vi "Actor Core.vi"(8 "error in (no error)":errorcluster, 11 "CalibrationManagerActor.lvlib:CalibrationManagerActor.lvclass":refnum<class "CalibrationManagerActor.lvclass">) -> (0 "error out":errorcluster, 3 "Actor out":refnum<class "Actor.lvclass">)   [LabVIEW 2017, in "CalibrationManagerActor.lvlib" / "CalibrationManagerActor.lvclass"]
doc: "This VI allows the user to view and edit instrument calibration details."
uses:
  CalibrationManagerActor.lvclass
  Library/SAM Resources 2.0/Main GUI/TSCalMan.llb/CalManData.ctl
  Library/SAM Resources 2.0/Main GUI/TSCalMan.llb/CalDataUnit.ctl
  <vilib>/ActorFramework/Actor/Actor.lvclass
  C:/Program Files (x86)/National Instruments/LabVIEW 2017/vi.lib/ActorFramework/Actor/Actor.lvclass
  SAMLite_DB/DB_Collections_class/mode.ctl
  CalibrationManagerActor.lvclass/CalibrationManagerActor.ctl
  Library/SAM Resources 2.0/Main GUI/TSCalMan.llb/CalMStates.ctl
  <vilib>/ActorFramework/Actor/Actor.lvclass/Actor.ctl
  <vilib>/ActorFramework/Message Enqueuer/Message Enqueuer.lvclass/Message Enqueuer.ctl
  <vilib>/ActorFramework/Message Enqueuer/Init from Existing Queue.vi
  <vilib>/ActorFramework/Message Enqueuer/Enqueue.vi
  <vilib>/ActorFramework/Stop Msg/Stop Msg.lvclass
  C:/Program Files (x86)/National Instruments/LabVIEW 2017/vi.lib/ActorFramework/Message/Message.lvclass
  <vilib>/ActorFramework/Message Priority Queue/Priority Enqueue.vi
  <vilib>/ActorFramework/Message Enqueuer/Message Enqueuer.lvclass
  GUI/GUI/GUI.lvclass
  Library/SAM Resources 2.0/Main GUI/SAMLite_Calibration Managemer.lvlib
  Library/SAM Resources 2.0/Main GUI/TestExec-STAC.llb/Full UI - Globals.vi
  Library/Amfax Library/Amfax Library/AmFax Source Code.lvclass
  SAMLite_DB/DB_Collections_class/DB_Collections.lvclass
  Library/Amfax Library/AmFax Source Code.lvlib
panel:
  in  "Edit Data File":bool
  in  "Calibration Data File":path
  in  "Alias Name":string
  out "Message":string
  in  "Cal Date Enabled":bool
  in  "Counter Enabled":bool
  in  "Calibration\n Interval":u32(ring) items=["Select an interval"=0, "1 month"=1, "2 months"=2, "6 months"=6, "12 months"=12, "24 months"=24]
  out "Current Count":u16=28 min=28 max=730 step=1
  in  "Total Cycles":i32
  in  "Cnt Warning":u16=28
  out "Traffic Light":cluster{"Red":bool, "Amber":bool, "Green":bool} caption="Calibration Status"
  in  "Reset Counter":bool
  in  "Cancel":bool
  in  "OK":bool
  in  "Cal Warning":u16=28
  in  "Type":string(combo)
  in  "Calibrated On":timestamp format="%<%x>T"
  in  "Cal Due Date":timestamp format="%<%x>T"
  in  "Cal":i32(listbox)
  out "Cal Expiry":u16=28 caption="Duration of\nCalibration" min=28 max=730 step=1
  in  "Clear All":bool
  in  "Delete":bool
  in  "Serial Number":string
  in  "Description":string
  in  "Update":bool
  in  "Add":bool
  in  "Cal Data FileName":string="CalInfo.bin"
  out "Cancelled":bool
  out "Calibration Out":T1 {"Cal Data Listing"."Cal Date" format="%<%x>T"; "Cal Data Listing"."Cal Due" format="%<%x>T"}
  out "Calibration Data Original":T1 {"Cal Data Listing"."Cal Date" format="%<%x>T"; "Cal Data Listing"."Cal Due" format="%<%x>T"}
  out "Out of Cal":bool
  # "Calibration Manager"
  # "Issue a Warning Message Ahead of Cycle Count by"
  # "Cycles"
  # "Days"
  # "Issue a Warning Message Ahead of Calibration Expiry Dates by"
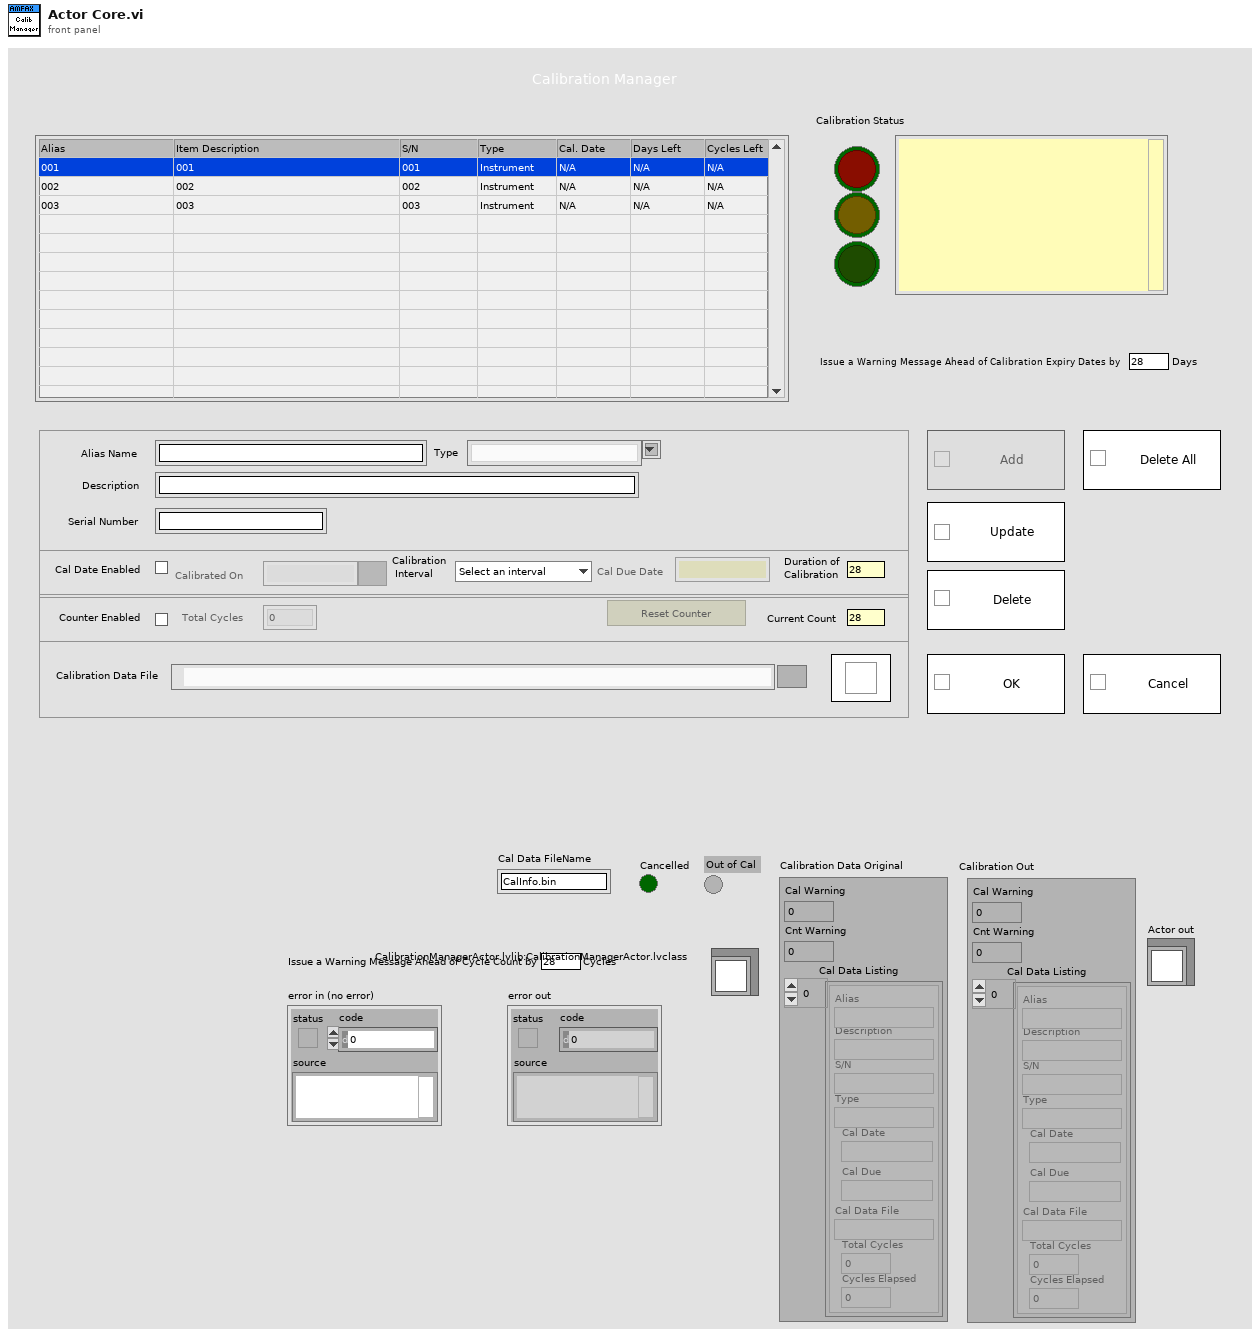
[diagram p1: front panel]
types:
  T1 = typedef "SAMLite_Calibration Managemer.lvlib/CalManData.ctl" = cluster{"Cal Warning":u32, "Cnt Warning":u16, "Cal Data Listing":T2[]}
  T2 = typedef "SAMLite_Calibration Managemer.lvlib/CalDataUnit.ctl" = cluster{"Alias":string, "Description":string, "S/N":string, "Type":string, "Cal Date":timestamp, "Cal Due":timestamp, "Cal Data File":path, "Total Cycles":i32, "Cycles Elapsed":i32}
  T3 = typedef "SAMLite_DB.lvlib/DB_Collections.lvclass/mode.ctl" = enum16{"read from file", "write to file", "set Defaults"}
  T4 = typedef "SAMLite_DB.lvlib/DB_Collections.lvclass/SAMLite Database.ctl" = cluster{"User Management":T5, "File Paths":cluster{"Path of test modules":path, "Path of sequences":path, "Path of test reports":path, "Path of Error Report":path, "Path of Calibration Data File":path, "Path of Company Logo":path, "Path of Startup VIs":path}, "Version Info":cluster{"Version No.":string}, "GUI Configuration":T8, "TARTCS_Intrument Control":T9, "Step Module Data":T17}
  T5 = typedef "SAMLite_DB.lvlib/DB_User.lvclass/User Management.ctl" = cluster{"Current User":string, "Current user group":T6, "Registered Users":cluster{"First Name":string, "Last Name":string, "User Name":string, "Password":string, "User Group":T6}[], "User Groups":cluster{"User Group":T6, "Members":string[], "User Previleges":T7}[]}
  T6 = typedef "SAMLite_DB.lvlib/DB_User.lvclass/User Group.ctl" = enum16{"Administrator", "Engineer", "Operator", "Data Viewer"}
  T7 = typedef "SAMLite_DB.lvlib/DB_User.lvclass/User Previleges.ctl" = cluster{"Run Sequences":bool, "Set Station Options":bool, "Instrument Configurations":bool, "Calibration Management":bool, "Access Test Reports Screen":bool, "Edit Test Sequences":bool, "Edit User":bool, "Add User":bool, "Delete User":bool, "Manual Control":bool, "Initialise System":bool}
  T8 = typedef "SAMLite_DB.lvlib/DB_SoftConfig.lvclass/GUI_Configurations.ctl" = cluster{"Main screen button caption color":u32, "Main screen display setting":enum32{"Modal", "Floating"}, "Debug Mode?":bool}
  T9 = typedef "SAMLite_DB.lvlib/DB_Collections.lvclass/TARTCS_InstrumentsSettings.ctl" = cluster{"Boom":T10, "Turntable":T13, "Inclinometer":T14, "Signal Generator Settings":cluster{"Resource Name (GPIB::28)":string}, "Spectrum Analyser Settings":cluster{"Resource Name (GPIB::28)":string}, "cRIO IP address":cluster{"Resource Name (GPIB::28)":string}}
  T10 = typedef "StreamComms.lvlib/Boom_Params.ctl" = cluster{"Master Node detail ":T11, "Slave Node Detail":T11, "Angle":dbl, "Motor Frequency %":dbl, "Max Leg Angle Difference":dbl, "Max Inclinometer to To Boom Leg  Angle Difference":dbl, "Angle Limits":cluster{"Max Operating Position":dbl, "Home Max Offset":dbl, "Home Position":dbl, "Home Min Offset":dbl, "Min Operating Position":dbl}, "Step Angle":dbl, "Select Boom/Inc Trigger":enum16{"Inclinometer", "Boom"}}
  T11 = typedef "StreamComms.lvlib/Inverter_NodeInfo.ctl" = cluster{"Node ID":u8, "baud rate":T12, "termination required? (F)":bool, "interface name":u32, "Inverter Name":string}
  T12 = typedef "CANopen BaudRate.ctl" = u32
  T13 = typedef "StreamComms.lvlib/Turntable_Params.ctl" = cluster{"Node Detail":T11, "Angle":dbl, "Motor Frequency %":dbl, "Trigger Step Angle":dbl}
  T14 = typedef "StreamComms.lvlib/Inclinometer_Params.ctl" = cluster{"Node Detail":T15, "filter cutoff (milli Hz)":dbl, "Triger angle":dbl, "Zero Offset (deg)":dbl}
  T15 = typedef "StreamComms.lvlib/CANOpen_NodeDetail.ctl" = cluster{"LSS Identity Details":T16, "Node ID":u8, "baud rate":T12, "termination required? (F)":bool, "interface name":u32}
  T16 = typedef "StreamComms.lvlib/CANOpen LSS Identity.ctl" = cluster{"Vendor ID":u32, "Product Code":u32, "Revision Number":u32, "Serial Number":u32}
  T17 = typedef "SAMLite_DB.lvlib/DB_StepModule.lvclass/Step Module Date.ctl" = cluster{"Error Out":errorcluster}
  T18 = enum8{"Enabled", "Disabled", "Disabled and Grayed Out"}
  T19 = typedef "CalibrationManagerActor.lvlib/CalibrationManagerActor.lvclass/CalMStates.ctl" = enum16{"Initialise", "Event", "Screen Update", "Save", "Exit"}
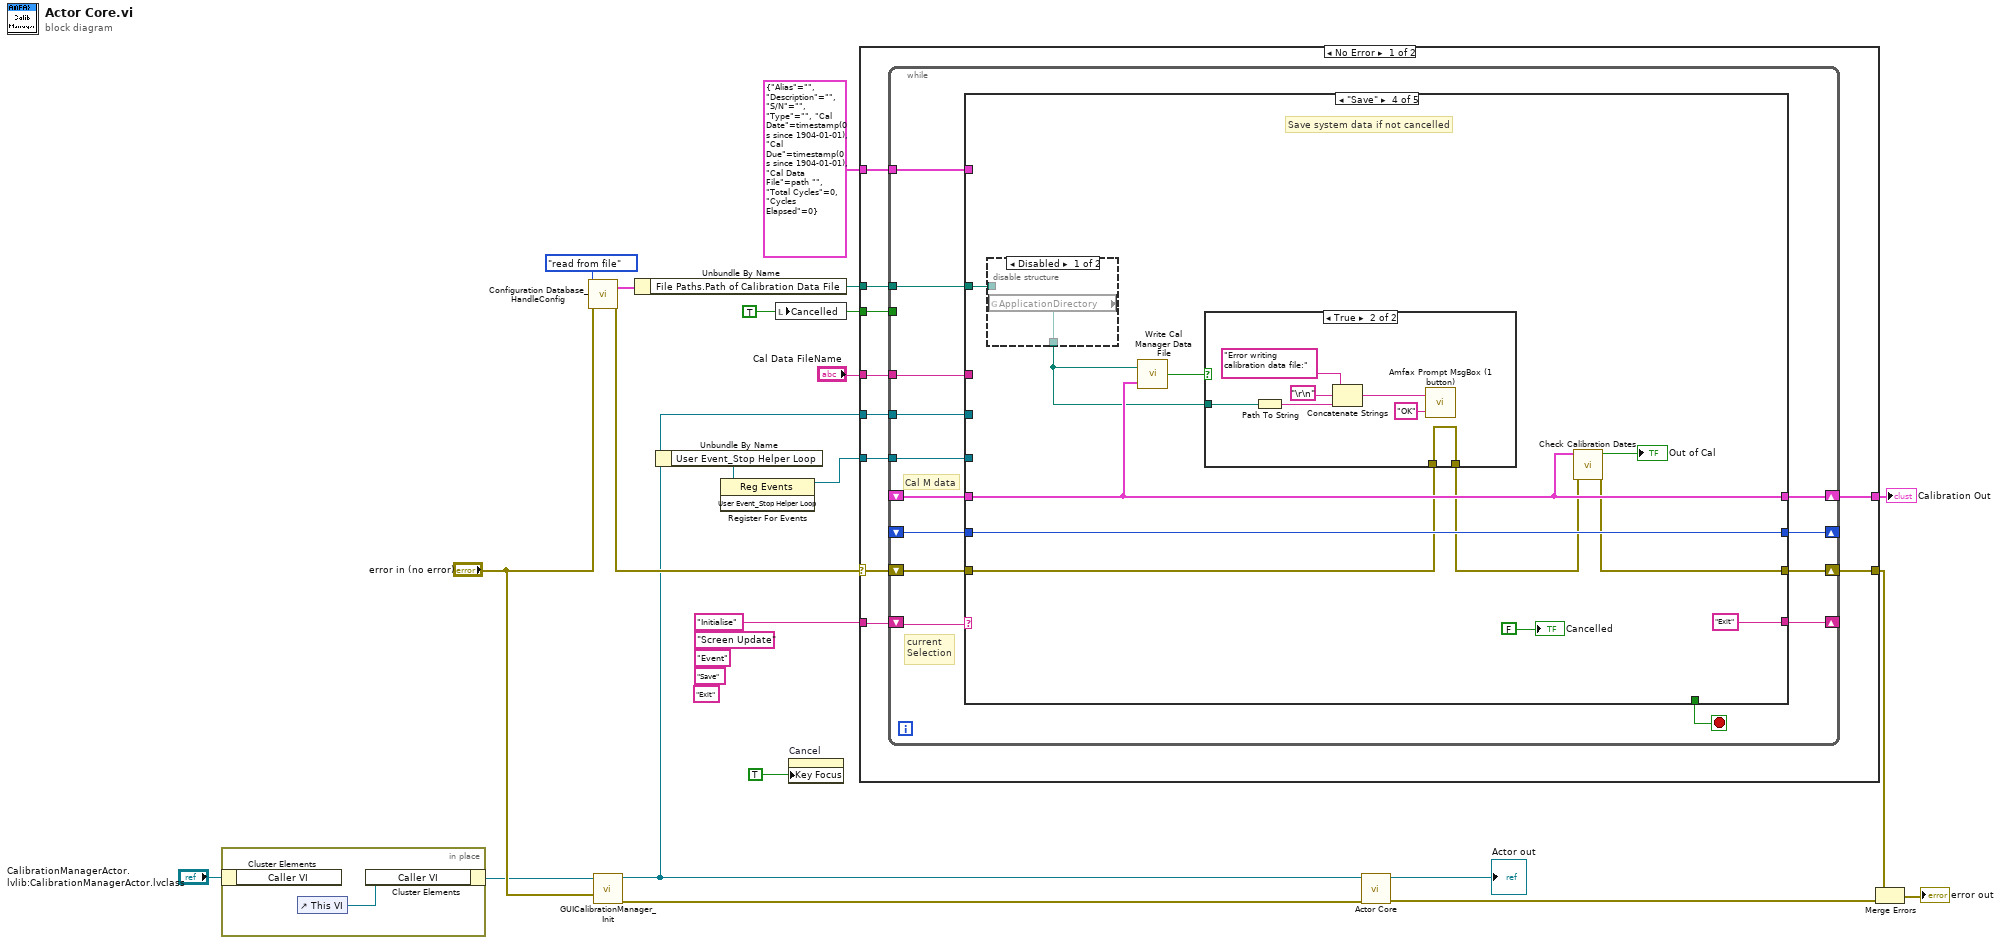
[diagram p0: block diagram]
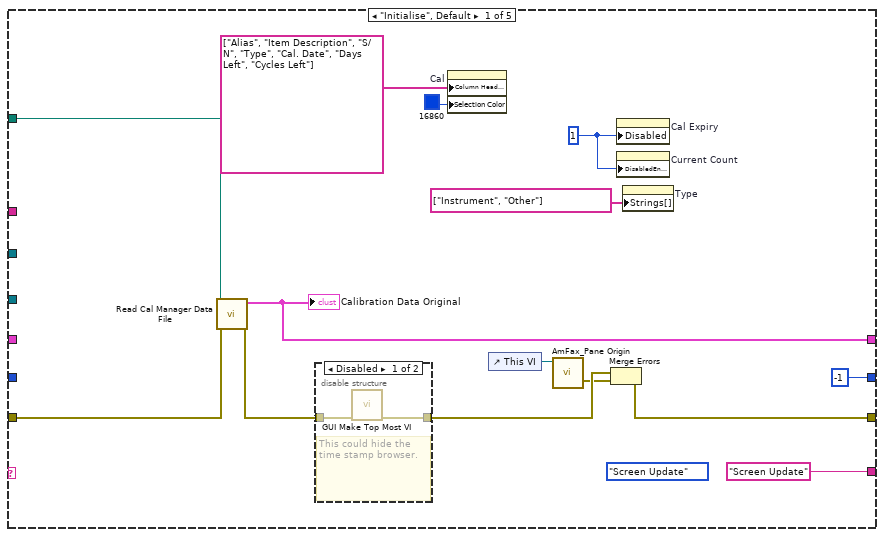
[diagram p2: hidden frame]
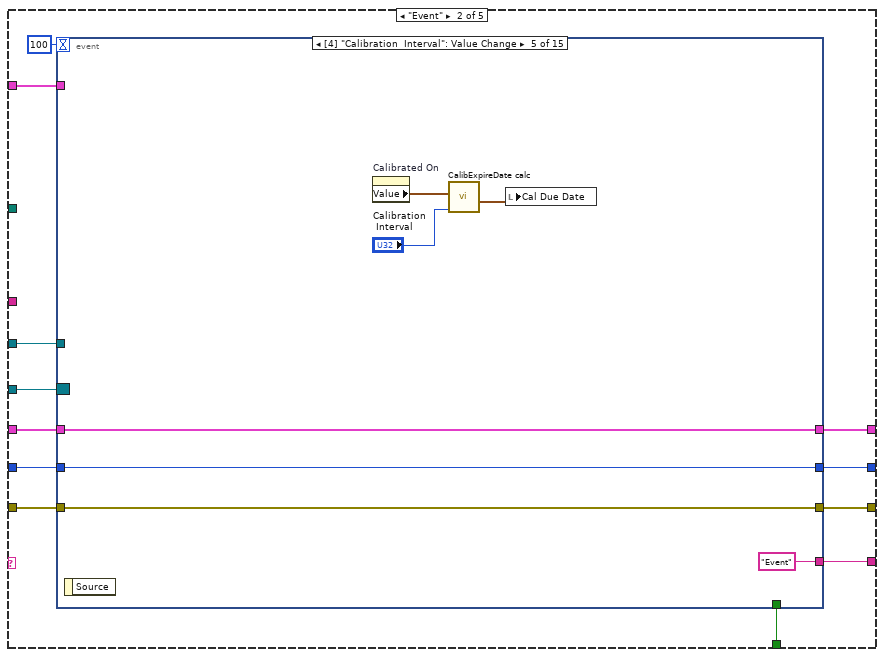
[diagram p4: hidden frame]
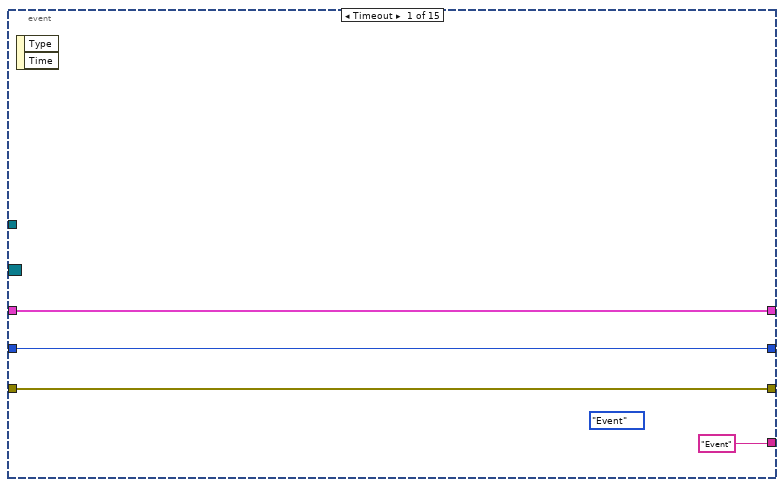
[diagram p5: hidden frame]
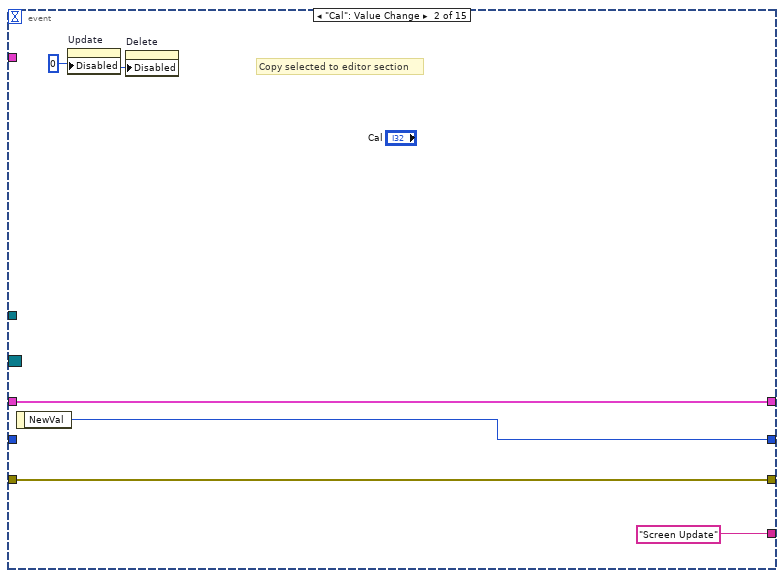
[diagram p6: hidden frame]
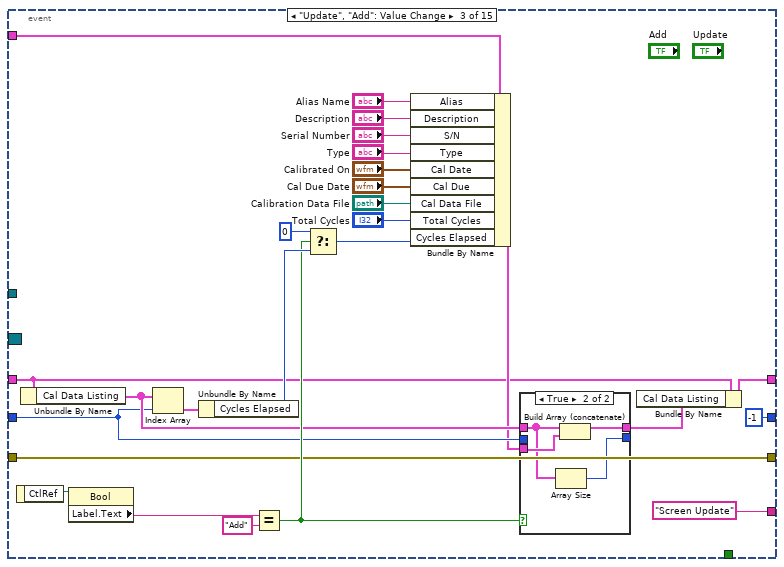
[diagram p7: hidden frame]
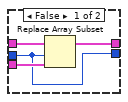
[diagram p8: hidden frame]
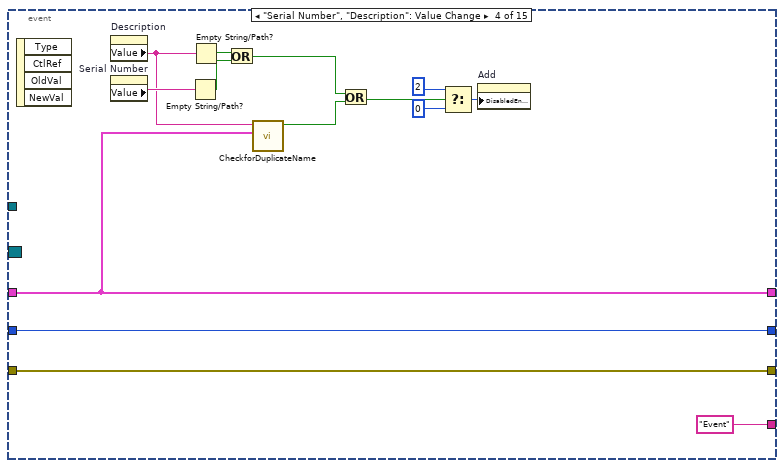
[diagram p9: hidden frame]
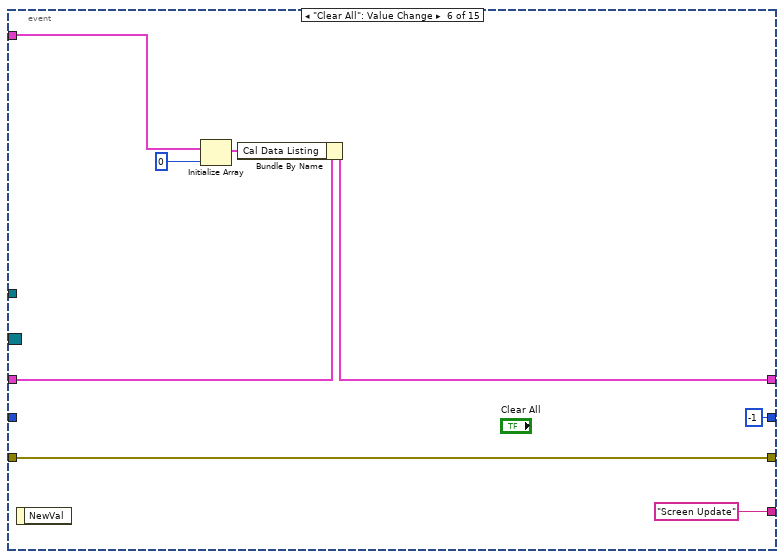
[diagram p10: hidden frame]
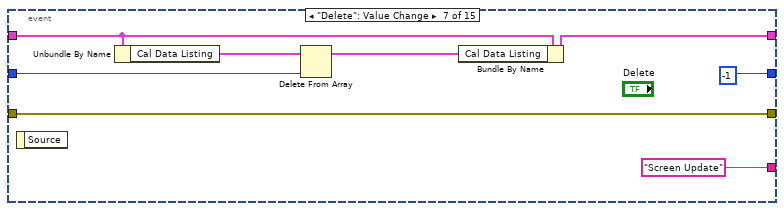
[diagram p11: hidden frame]
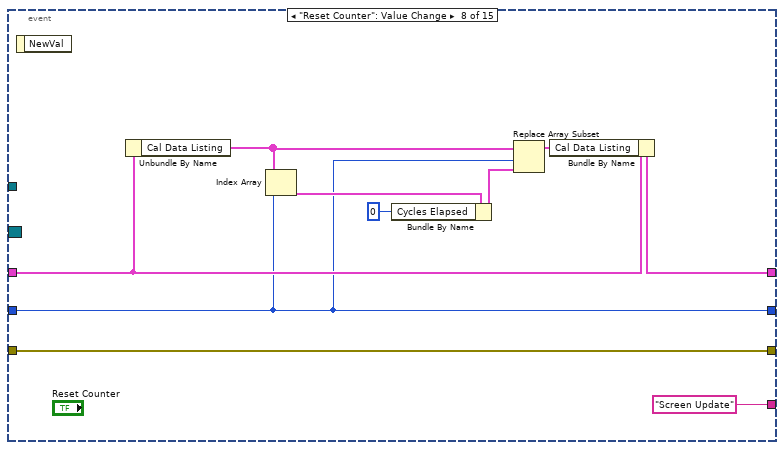
[diagram p12: hidden frame]
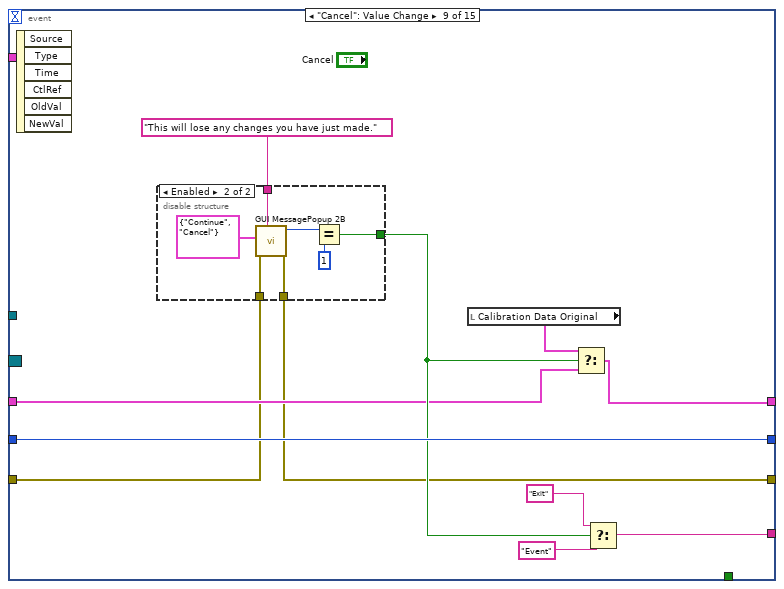
[diagram p13: hidden frame]
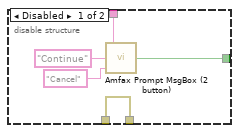
[diagram p14: hidden frame]
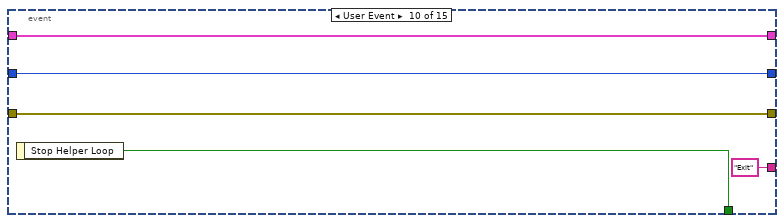
[diagram p15: hidden frame]
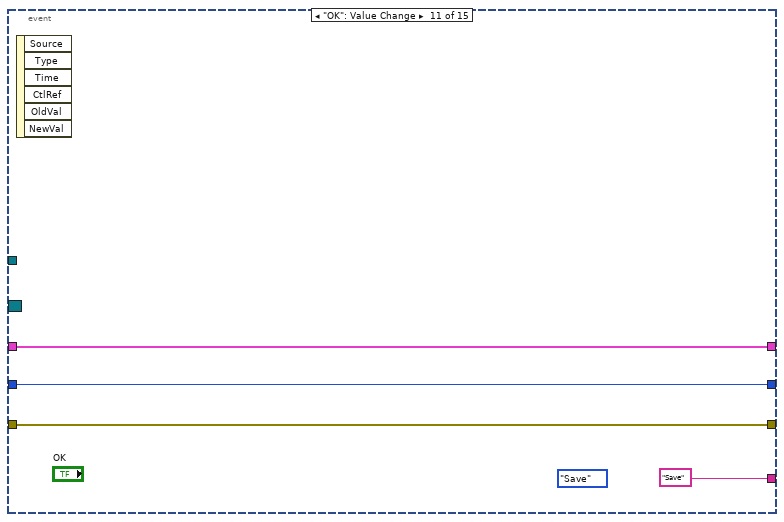
[diagram p16: hidden frame]
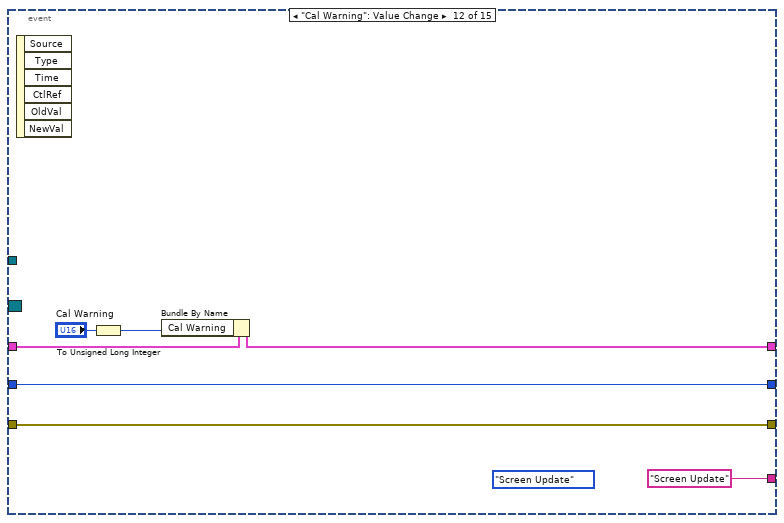
[diagram p17: hidden frame]
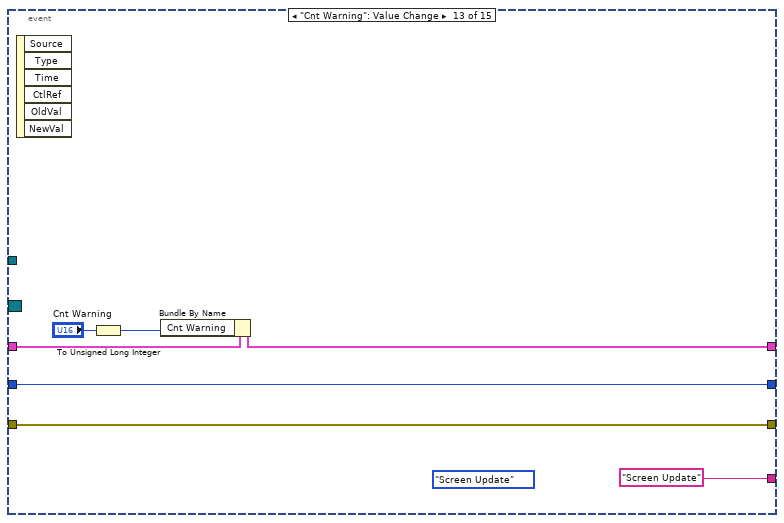
[diagram p18: hidden frame]
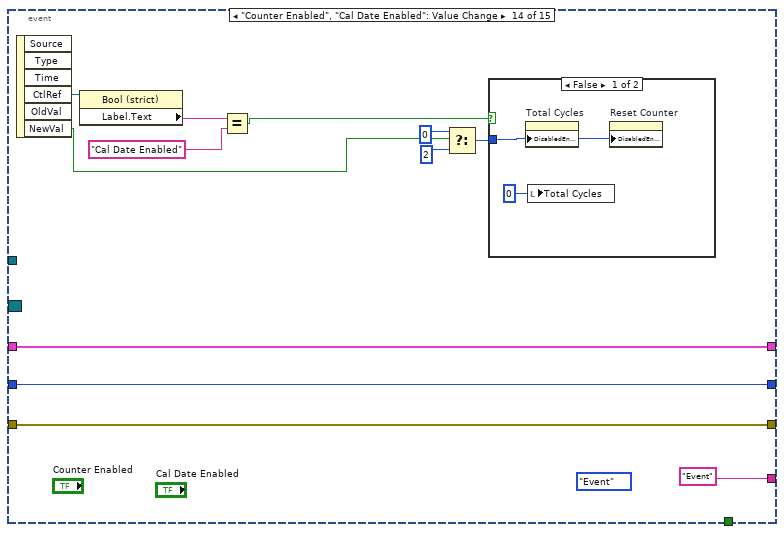
[diagram p19: hidden frame]
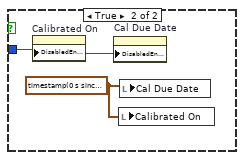
[diagram p20: hidden frame]
diagram:
  (unwired) "Screen Update"
  (unwired) "Exit"
  (unwired) "Save"
  (unwired) "Event"
  w19 = TRUE ("Cancelled")
  n1 = in-place {
    n2 = in-place-cluster #1("CalibrationManagerActor.lvlib:CalibrationManagerActor.lvclass") -> ()  [unwired: 1 out]
    n3 = control-ref of="This VI"() -> (w22:refnum<vi>)
    n4 = in-place-cluster #1("Caller VI"=w22) -> (w1:refnum<class "CalibrationManagerActor.lvclass">)
  }
  n5 = call "Configuration Database_HandleConfig.vi"("error in (no error)"="error in (no error)", "Task"=mode."read from file") -> ("error out"=w13:errorcluster, "SAMLite Database  out"=w16:T4)  [unwired: 8 in]
  n6 = call "GUICalibrationManager_Init.vi"("error in (no error)"="error in (no error)", "GUI_About in"=w1) -> ("error out"=w6:errorcluster, "GUI_About out"=w5:refnum<class "CalibrationManagerActor.lvclass">)  [unwired: 8 in]
  n7 = Unbundle By Name(w16) -> ("File Paths.Path of Calibration Data File"=w14:path)
  n8 = Unbundle By Name(w5) -> ("User Event_Stop Helper Loop"=w4:refnum<user-event>)
  n9 = register-events(w4) -> (reference out=w3:refnum<event-registration>)  [unwired: 2 in, 1 out]
  n10 = local write "Cancelled"(w19) -> ()
  n11 = property on="Cancel" class="Bool"("Key Focus"=TRUE) -> ()  [unwired: 2 in, 2 out]
  n12 = case shown="No Error" w13 {
    selector: w13 -> [w27 w339]
    tunnel: "Cal Data FileName" -> [w32 _]
    tunnel: "Initialise" -> [w31 _]
    tunnel: w19 -> [w30 _]
    tunnel: T2 {"Alias"="", "Description"="", "S/N"="", "Type"="", "Cal Date"=timestamp(0 s since 1904-01-01), "Cal Due"=timestamp(0 s since 1904-01-01), "Cal Data File"=path "", "Total Cycles"=0, "Cycles Elapsed"=0} -> [w29 _]
    tunnel: [w28 T1 {"Cal Warning"=0, "Cnt Warning"=0, "Cal Data Listing"=[]} ("Calibration Data Original")] -> w17
    tunnel: [w26 w339] -> w11
    tunnel: w14 -> [w25 _]
    tunnel: w5 -> [w24 _]
    tunnel: w3 -> [w23 _]
    frame No Error {
      n13 = while {
        shift-left: _ -> [w46]
        shift-right: [w44] -> w28
        shift-right: [w41] -> _
        shift-left: w31 -> [w43]
        tunnel: w32 -> [w42]
        tunnel: w30 -> [_]
        shift-right: [w40] -> _
        shift-left: _ -> [w39]
        tunnel: w29 -> [w38]
        shift-right: [w36] -> w26
        shift-left: w27 -> [w37]
        tunnel: w25 -> [w35]
        tunnel: w24 -> [w34]
        tunnel: w23 -> [w33]
        stop <- w45 stop-if-true
        # "current\nSelection"
        # "Cal M data"
        n14 = case shown="\"Save\"" w43 {
          tunnel: w46 -> [_ w75 w245 w316 w337]
          tunnel: [_ w64 _ _ TRUE ("T button?")] -> w45
          tunnel: [w55 w74 w245 w316 w337] -> w44
          tunnel: w42 -> [_ _ _ _ _]
          tunnel: ["Screen Update" w72 "Event" "Exit" "Exit"] -> w41
          tunnel: [-1 ("NewVal") w71 w270 w313 w335] -> w40
          tunnel: w39 -> [_ w69 w270 w313 w335]
          tunnel: w38 -> [_ w70 _ _ _]
          tunnel: w37 -> [w54 w68 w242 w312 w329]
          tunnel: [w49 w67 w242 w310 w334] -> w36
          tunnel: w35 -> [w48 _ w241 w309 _]
          tunnel: w34 -> [_ w66 _ _ w331]
          tunnel: w33 -> [_ w65 _ _ _]
          frame "Initialise", Default {
            w57 = u8 1 ("Disabled")
            (unwired) CalMStates."Screen Update" ("CalManState")
            n15 = call "Read Cal Manager Data File.vi"("error in (no error)"=w54, "Calibration File"=w48) -> ("Error Out"=w53:errorcluster, "Calibration Data"=w55:T1)  [unwired: 8 in]
            "Calibration Data Original" <- w55
            n16 = disable-structure shown="Disabled" {
              disable-tunnel: w53 -> [w62 w63]
              disable-tunnel: [w61 w63] -> w51
              frame Disabled {
                # "This could hide the time stamp browser."
                n17 = call "GUI Make Top Most VI.vi"("error in"=w62) -> ("error out"=w61:errorcluster)  [unwired: 10 in]
              }
              frame Enabled {
              }
            }
            n18 = property on="Cal" class="MCListbox (strict)"("Column Header Strings[]"=string[] ["Alias", "Item Description", "S/N", "Type", "Cal. Date", "Days Left", "Cycles Left"] ("Column Headers[]"), "Selection Color"=u32 16860) -> ()  [unwired: 2 in, 2 out]
            n19 = control-ref of="This VI"() -> (w52:refnum<vi>)
            n20 = call "AmFax_Pane Origin.vi"("This VI"=w52) -> ("error out"=w50:errorcluster)  [unwired: 9 in, 1 out]
            n21 = Merge Errors(w51, w50) -> (w49:errorcluster)
            n22 = property on="Cal Expiry" class="DigNum (strict)"("Disabled"=w57) -> ()  [unwired: 2 in, 2 out]
            n23 = property on="Current Count" class="DigNum (strict)"("DisabledEnum"=w57) -> ()  [unwired: 2 in, 2 out]
            n24 = property on="Type" class="CmbBox"("Strings[]"=string[] ["Instrument", "Other"] ("Strings []")) -> ()  [unwired: 2 in, 2 out]
          }
          frame "Event" {
            n25 = event shown="[4] \"Calibration  Interval\": Value Change" {
              selector: w65 -> [_ _ _ _ _ _ _ _ _ _ _ _ _ _ _]
              dyn-events: _ -> [_ _ _ _ _ _ _ _ _ _ _ _ _ _ _]
              timeout: 100 -> [_ _ _ _ _ _ _ _ _ _ _ _ _ _ _]
              tunnel: w75 -> [w79 w83 w92 w131 w137 w146 w155 w159 w173 w189 w197 w202 w210 w220 w236]
              tunnel: [w79 w83 w91 w131 w137 w147 w154 w160 w172 w189 w197 w201 w209 w220 w236] -> w74
              tunnel: ["Event" "Screen Update" "Screen Update" "Event" "Event" "Screen Update" "Screen Update" "Screen Update" w176 "Exit" "Save" "Screen Update" "Screen Update" "Event" "Screen Update"] -> w72
              tunnel: [w78 w82 -1 ("Cal") w132 w138 -1 ("NewVal") -1 ("Cal") w158 w175 w190 w196 w200 w207 w219 w237] -> w71
              tunnel: w70 -> [_ _ w110 _ _ w145 _ _ _ _ _ _ _ _ _]
              tunnel: w69 -> [w78 _ w94 w132 w138 _ w150 w158 w175 w190 w196 w200 w207 w219 w237]
              tunnel: w68 -> [w77 w81 w86 w120 w134 w141 w149 w157 w170 w191 w195 w199 w206 w213 w231]
              tunnel: [w77 w81 w86 w120 w134 w141 w149 w157 w169 w191 w195 w199 w206 w213 w230] -> w67
              tunnel: w66 -> [_ _ _ _ _ _ _ _ _ _ _ _ _ _ _]
              tunnel: [_ _ _ _ _ _ _ _ _ w193 _ _ _ _ _] -> w64
              event Timeout {
                (unwired) CalMStates."Event" ("CalManState")
                n26 = event-data() -> ()  [unwired: 1 in, 2 out]
              }
              event "Cal": Value Change {
                w84 = u8 0
                # "Copy selected to editor section"
                n27 = event-data() -> ("NewVal"=w82:i32)  [unwired: 1 in]
                n28 = property on="Update" class="Bool"("Disabled"=w84) -> ()  [unwired: 2 in, 2 out]
                n29 = property on="Delete" class="Bool"("Disabled"=w84) -> ()  [unwired: 2 in, 2 out]
              }
              event "Update", "Add": Value Change {
                n30 = event-data() -> ("CtlRef"=w101:refnum<vi>)  [unwired: 1 in]
                n31 = Unbundle By Name(w92) -> ("Cal Data Listing"=w95:T2[])
                n32 = property class="Bool"(reference=w101) -> ("Label.Text"=w100:string)  [unwired: 1 in, 2 out]
                n33 = Index Array(array=w95, index=w94) -> (element=w98:T2)
                n34 = Unbundle By Name(w98) -> ("Cycles Elapsed"=w97:i32)
                n35 = Equal?(x=w100, y="Add") -> (x = y?=w96:bool)
                n36 = Select(t=0 ("Cycles Elapsed"), s=w96, f=w97) -> (s? t:f=w102:i32)
                n37 = Bundle By Name(cluster=w110, "Alias"="Alias Name", "Description"="Description", "S/N"="Serial Number", "Type"="Type", "Cal Date"="Calibrated On", "Cal Due"="Cal Due Date", "Cal Data File"="Calibration Data File", "Total Cycles"="Total Cycles", "Cycles Elapsed"=w102) -> (w93:T2)
                n38 = case shown="True" w96 {
                  tunnel: w95 -> [w114 w116]
                  tunnel: w94 -> [w111 _]
                  tunnel: w93 -> [w113 w118]
                  tunnel: [w112 w117] -> w90
                  tunnel: [w111 w115] -> _
                  frame False {
                    n39 = Replace Array Subset(array=w114, new element=w113, index=w111) -> (w112:T2[])
                  }
                  frame True {
                    n40 = Array Size(array=w116) -> (size(s)=w115:i32)
                    n41 = Build Array (concatenate)(w116, w118) -> (w117:T2[])
                  }
                }
                n42 = Bundle By Name(cluster=w92, "Cal Data Listing"=w90) -> (w91:T1)
              }
              event "Serial Number", "Description": Value Change {
                n43 = event-data() -> ()  [unwired: 1 in, 4 out]
                n44 = property on="Description" class="Str"() -> ("Value"=w121:string)  [unwired: 2 in, 2 out]
                n45 = property on="Serial Number" class="Str"() -> ("Value"=w130:string)  [unwired: 2 in, 2 out]
                n46 = Empty String/Path?(string/path=w130) -> (empty?=w128:bool)
                n47 = Empty String/Path?(string/path=w121) -> (empty?=w129:bool)
                n48 = Or(x=w129, y=w128) -> (x .or. y?=w127:bool)
                n49 = call "CheckforDuplicateName.vi"("Calibration Data"=w131, "Alias"=w121) -> ("Duplicate Found"=w122:bool)  [unwired: 9 in]
                n50 = Or(x=w127, y=w122) -> (x .or. y?=w124:bool)
                n51 = Select(t=2, s=w124, f=0) -> (s? t:f=w123:i32)
                n52 = property on="Add" class="Bool"("DisabledEnum"=w123) -> ()  [unwired: 2 in, 2 out]
              }
              event "Calibration\n Interval": Value Change {
                n53 = event-data() -> ()  [unwired: 1 in, 1 out]
                n54 = property on="Calibrated On" class="AbsTime (strict)"() -> ("Value"=w135:timestamp)  [unwired: 2 in, 2 out]
                n55 = call "CalibExpireDate calc.vi"("Calibration Interval"="Calibration\n Interval", "Calibration Date"=w135) -> ("Calibration Expire"=w136:timestamp)  [unwired: 9 in]
                n56 = local write "Cal Due Date"(w136) -> ()
              }
              event "Clear All": Value Change {
                n57 = event-data() -> ()  [unwired: 1 in, 1 out]
                n58 = Initialize Array(w145, 0 ("dimension size")) -> (w143:T2[])
                n59 = Bundle By Name(cluster=w146, "Cal Data Listing"=w143) -> (w147:T1)
              }
              event "Delete": Value Change {
                n60 = event-data() -> ()  [unwired: 1 in, 1 out]
                n61 = Unbundle By Name(w155) -> ("Cal Data Listing"=w153:T2[])
                n62 = Delete From Array(array=w153, index=w150) -> (array with subset deleted=w152:T2[])  [unwired: 1 in, 1 out]
                n63 = Bundle By Name(cluster=w155, "Cal Data Listing"=w152) -> (w154:T1)
              }
              event "Reset Counter": Value Change {
                n64 = event-data() -> ()  [unwired: 1 in, 1 out]
                n65 = Unbundle By Name(w159) -> ("Cal Data Listing"=w163:T2[])
                n66 = Index Array(array=w163, index=w158) -> (element=w165:T2)
                n67 = Bundle By Name(cluster=w165, "Cycles Elapsed"=0) -> (w162:T2)
                n68 = Replace Array Subset(array=w163, new element=w162, index=w158) -> (w161:T2[])
                n69 = Bundle By Name(cluster=w159, "Cal Data Listing"=w161) -> (w160:T1)
              }
              event "Cancel": Value Change {
                n70 = event-data() -> ()  [unwired: 1 in, 6 out]
                n71 = disable-structure shown="Enabled" {
                  disable-tunnel: [w179 w182] -> w174
                  disable-tunnel: w170 -> [w177 w188]
                  disable-tunnel: [w177 w187] -> w169
                  disable-tunnel: "This will lose any changes you have just made." -> [w178 w186]
                  frame Disabled {
                    n72 = call "Amfax Prompt MsgBox (2 button).vi"("Right button name"="Cancel" ("F button name (\"Cancel\")"), "Left button name"="Continue" ("T button name (\"OK\")"), "Message"=w178) -> ("Left Button?"=w179:bool)
                  }
                  frame Enabled {
                    n73 = call "GUI MessagePopup 2B.vi"("Message"=w186, "error in"=w188, "Info"=cluster{"Control1":string, "Control2":string} {"Control1"="Continue", "Control2"="Cancel"}) -> ("error out"=w187:errorcluster, "ButtonPressed"=w184:u16)  [unwired: 7 in]
                    n74 = Equal?(x=w184, y=u16 1) -> (x = y?=w182:bool)
                  }
                }
                n75 = local read "Calibration Data Original"() -> (w171:T1)
                n76 = Select(t=w171, s=w174, f=w173) -> (s? t:f=w172:T1)
                n77 = Select(t="Exit", s=w174, f="Event") -> (s? t:f=w176:string)
              }
              event User Event {
                n78 = event-data() -> ("Stop Helper Loop"=w193:bool)  [unwired: 1 in]
              }
              event "OK": Value Change {
                (unwired) CalMStates."Save" ("CalManState")
                n79 = event-data() -> ()  [unwired: 1 in, 6 out]
              }
              event "Cal Warning": Value Change {
                (unwired) CalMStates."Screen Update" ("CalManState")
                n80 = event-data() -> ()  [unwired: 1 in, 6 out]
                n81 = To Unsigned Long Integer(number="Cal Warning") -> (unsigned 32bit integer=w203:u32)
                n82 = Bundle By Name(cluster=w202, "Cal Warning"=w203) -> (w201:T1)
              }
              event "Cnt Warning": Value Change {
                (unwired) CalMStates."Screen Update" ("CalManState")
                n83 = event-data() -> ()  [unwired: 1 in, 6 out]
                n84 = To Unsigned Long Integer(number="Cnt Warning") -> (unsigned 32bit integer=w211:u32)
                n85 = Bundle By Name(cluster=w210, "Cnt Warning"=w211) -> (w209:T1)
              }
              event "Counter Enabled", "Cal Date Enabled": Value Change {
                (unwired) CalMStates."Event" ("CalManState")
                n86 = event-data() -> ("CtlRef"=w223:refnum<vi>, "NewVal"=w215:bool)  [unwired: 1 in, 4 out]
                n87 = property class="Bool (strict)"(reference=w223) -> ("Label.Text"=w222:string)  [unwired: 1 in, 2 out]
                n88 = Equal?(x=w222, y="Cal Date Enabled") -> (x = y?=w216:bool)
                n89 = Select(t=0, s=w215, f=2) -> (s? t:f=w217:i32)
                n90 = case shown="False" w216 {
                  tunnel: w217 -> [w225 w226]
                  frame False {
                    n91 = property on="Total Cycles" class="DigNum (strict)"("DisabledEnum"=w225) -> ()  [unwired: 2 in, 2 out]
                    n92 = local write "Total Cycles"(0 ("Total Cycles")) -> ()
                    n93 = property on="Reset Counter" class="Bool"("DisabledEnum"=w225) -> ()  [unwired: 2 in, 2 out]
                  }
                  frame True {
                    w227 = timestamp(0 s since 1904-01-01) ("Cal Due Date")
                    n94 = property on="Calibrated On" class="AbsTime (strict)"("DisabledEnum"=w226) -> ()  [unwired: 2 in, 2 out]
                    n95 = property on="Cal Due Date" class="AbsTime (strict)"("DisabledEnum"=w226) -> ()  [unwired: 2 in, 2 out]
                    n96 = local write "Calibrated On"(w227) -> ()
                    n97 = local write "Cal Due Date"(w227) -> ()
                  }
                }
              }
              event "Edit Data File": Value Change {
                (unwired) CalMStates."Screen Update" ("CalManState")
                n98 = event-data() -> ()  [unwired: 1 in, 1 out]
                n99 = Unbundle By Name(w236) -> ("Cal Data Listing"=w238:T2[])
                n100 = Index Array(array=w238, index=w237) -> (element=w239:T2)
                n101 = Unbundle By Name(w239) -> ("Cal Data File"=w235:path)
                n102 = Format Into String(format string="notepad %s", error in=w231, w235) -> (resulting string=w233:string, error out=w232:errorcluster)  [unwired: 1 in]
                n103 = call <vilib>:"System Exec.vi"("wait until completion? (T)"=FALSE, "error in (no error)"=w232, "command line"=w233) -> ("error out"=w230:errorcluster)  [unwired: 5 in, 3 out]
              }
            }
          }
          frame "Screen Update" {
            w264 = 2
            w265 = 0
            n104 = Less Than 0?(x=w270) -> (x < 0?=w281:bool)
            n105 = case shown="False" w281 {
              tunnel: w245 -> [w298 _]
              tunnel: w270 -> [w296 _]
              tunnel: [w294 w300] -> w247
              tunnel: [w293 w300] -> w253
              tunnel: [w292 w306] -> w244
              tunnel: [w291 w305] -> w262
              tunnel: [w290 w305] -> w260
              tunnel: [w289 path ""] -> w280
              tunnel: [w288 w304] -> w268
              tunnel: [w287 w304] -> w279
              tunnel: [T18."Enabled" ("Disabled") T18."Disabled and Grayed Out" ("Disabled")] -> w271
              tunnel: [w284 u32 0 ("Calibration Interval")] -> w269
              tunnel: [w285 w300] -> w243
              tunnel: w241 -> [_ _]
              frame False {
                w284 = u32 0 items=["Select an interval"=0, "1 month"=1, "2 months"=2, "6 months"=6, "12 months"=12, "24 months"=24] ("Calibration\n Interval")
                n106 = Unbundle By Name(w298) -> ("Cal Data Listing"=w297:T2[])
                n107 = Index Array(array=w297, index=w296) -> (element=w295:T2)
                n108 = Unbundle By Name(w295) -> ("Alias"=w285:string, "Description"=w294:string, "S/N"=w293:string, "Type"=w292:string, "Cal Date"=w291:timestamp, "Cal Due"=w290:timestamp, "Cal Data File"=w289:path, "Total Cycles"=w288:i32, "Cycles Elapsed"=w287:i32)
              }
              frame True {
                w304 = 0 ("Total Cycles")
                w305 = timestamp(0 s since 1904-01-01)
                w300 = ""
                n109 = property on="Type" class="CmbBox"() -> ("Strings[]"=w301:string[])  [unwired: 2 in, 2 out]
                n110 = Index Array(array=w301) -> (element=w306:string)  [unwired: 1 in]
              }
            }
            "Current Count" <- w279
            n111 = Unbundle By Name(w245) -> ("Cal Warning"=w274:u32, "Cnt Warning"=w272:u16)
            n112 = property on="Cal" class="MCListbox (strict)"("Value"=w270) -> ()  [unwired: 2 in, 2 out]
            n113 = To Unsigned Word Integer(number=w274) -> (unsigned 16bit integer=w273:u16)
            n114 = local write "Cnt Warning"(w272) -> ()
            n115 = local write "Cal Warning"(w273) -> ()
            n116 = Get Date/Time In Seconds() -> (seconds since 1Jan1904=w278:timestamp)
            n117 = local write "Description"(w247) -> ()
            n118 = local write "Alias Name"(w243) -> ()
            n119 = local write "Calibration Data File"(w280) -> ()
            n120 = local write "Serial Number"(w253) -> ()
            n121 = local write "Type"(w244) -> ()
            n122 = local write "Calibration\n Interval"(w269) -> ()
            n123 = Subtract(x=w260, y=w278) -> (x-y=w277:dbl)
            n124 = local write "Cal Due Date"(w260) -> ()
            n125 = local write "Calibrated On"(w262) -> ()
            n126 = local write "Total Cycles"(w268) -> ()
            n127 = Divide(x=w277, y=u32 86400) -> (x/y=w275:dbl)
            n128 = property on="Update" class="Bool"("Disabled"=w271) -> ()  [unwired: 2 in, 2 out]
            n129 = property on="Delete" class="Bool"("Disabled"=w271) -> ()  [unwired: 2 in, 2 out]
            n130 = Empty String/Path?(string/path=w253) -> (empty?=w252:bool)
            n131 = call "CheckforDuplicateName.vi"("Calibration Data"=w245, "Alias"=w243) -> ("Duplicate Found"=w246:bool)  [unwired: 9 in]
            n132 = To Unsigned Word Integer(number=w275) -> (unsigned 16bit integer=w259:u16)
            n133 = Not Equal To 0?(x=w268) -> (x != 0?=w266:bool)
            n134 = Not Equal?(x=w262, y=timestamp(0 s since 1904-01-01) ("Cal Due Date")) -> (x != y?=w256:bool)
            n135 = local write "Counter Enabled"(w266) -> ()
            n136 = local write "Cal Date Enabled"(w256) -> ()
            n137 = Select(t=u16 0, s=w256, f=w259) -> (s? t:f=→"Cal Expiry":u16)
            n138 = Select(t=w265, s=w266, f=w264) -> (s? t:f=w263:i32)
            n139 = Select(t=w265, s=w256, f=w264) -> (s? t:f=w261:i32)
            n140 = Compound Arithmetic op=OR(w246, w252) -> (w250:bool)
            n141 = property on="Calibrated On" class="AbsTime (strict)"("DisabledEnum"=w261) -> ()  [unwired: 2 in, 2 out]
            n142 = property on="Total Cycles" class="DigNum (strict)"("DisabledEnum"=w263) -> ()  [unwired: 2 in, 2 out]
            n143 = Select(t=2, s=w250, f=0) -> (s? t:f=w248:i32)
            n144 = property on="Reset Counter" class="Bool"("DisabledEnum"=w263) -> ()  [unwired: 2 in, 2 out]
            n145 = property on="Cal Due Date" class="AbsTime (strict)"("DisabledEnum"=w261) -> ()  [unwired: 2 in, 2 out]
            n146 = call "Update Cal Manager Table.vi"("Calibration Data"=w245) -> ("Cal Table"=w283:string[][])  [unwired: 1 in]
            n147 = call "Check Calibration Dates.vi"("Calibration Data"=w245) -> ("Message Out"=→"Message":string, "Status"=w255:u16)  [unwired: 7 in, 2 out]
            n148 = property on="Add" class="Bool"("DisabledEnum"=w248) -> ()  [unwired: 2 in, 2 out]
            n149 = call "trafficlight.vi"("Status"=w255) -> ("Traffic Light"=→"Traffic Light":cluster{"Red":bool, "Amber":bool, "Green":bool})  [unwired: 7 in]
            n150 = property on="Cal" class="MCListbox (strict)"("Item Names"=w283) -> ()  [unwired: 2 in, 2 out]
          }
          frame "Save" {
            # "Save system data if not cancelled"
            n151 = disable-structure shown="Disabled" {
              disable-tunnel: [w318 w319] -> w308
              disable-tunnel: w309 -> [_ w319]
              frame Disabled {
                n152 = global read "Full UI - Globals.vi" "ApplicationDirectory"() -> (w318:path)
              }
              frame Enabled {
              }
            }
            n153 = call "Write Cal Manager Data File.vi"("Calibration Data"=w316, "Calibration File"=w308) -> ("Error"=w317:bool)
            n154 = case shown="True" w317 {
              tunnel: w308 -> [_ w326]
              tunnel: w312 -> [w320 w322]
              tunnel: [w320 w322] -> w311
              frame False {
              }
              frame True {
                n155 = Path To String(path=w326) -> (string=w325:string)
                n156 = Concatenate Strings("Error writing calibration data file:", "\r\n", w325) -> (w323:string)
                n157 = call "Amfax Prompt MsgBox (1 button).vi"("Middle button name"="OK", "Message"=w323) -> ()  [unwired: 1 out]
              }
            }
            n158 = call "Check Calibration Dates.vi"("error in (no error)"=w311, "Calibration Data"=w316) -> ("error out"=w310:errorcluster, "Out of Cal"=→"Out of Cal":bool)  [unwired: 6 in, 2 out]
            "Cancelled" <- FALSE ("Cancelled")
          }
          frame "Exit" {
            w333 = TRUE  # Close Window?
            n159 = call <vilib>:"Read Self Enqueuer.vi"("Actor"=w331) -> ("Self Enqueuer"=w330:refnum<class "Message Enqueuer.lvclass">)  [unwired: 10 in]
            n160 = call <vilib>:"Send Normal Stop.vi"("error in (no error)"=w329, "Message Enqueuer"=w330) -> ("error out"=w328:errorcluster)  [unwired: 9 in]
            n161 = call "GUI Make Top Most VI.vi"("error in"=w328, "Close Window?"=w333) -> ("error out"=w334:errorcluster)  [unwired: 9 in]
          }
        }
      }
    }
    frame Error {
    }
  }
  "Calibration Out" <- w17
  n162 = call-parent "Actor Core.vi"("error in"=w6, "Actor in"=w5) -> ("error out"=w10:errorcluster, "Actor out"=→"Actor out":refnum<class "Actor.lvclass">)  [unwired: 8 in]
  n163 = Merge Errors(w11, w10) -> (→"error out":errorcluster)
